vi "Test CAN Flatten.vi"() -> ()   [LabVIEW 2021]
uses:
  typedef/Datatype CAN.ctl
  CIFfifo.lvclass
  CIFfifo.lvclass/CIFfifo.ctl
  Utilities/Flatten Header.vi
  Flatten/CAN Flatten.vi/be899675-9489-4ae7-9bdb-bbc908cd9623.vi
  Flatten/CAN Flatten.vi/fa4e04b0-1c28-4039-87e0-9391600efeb5.vi
  Flatten/CAN Flatten.vi/24dfac9c-4f7b-471b-adb6-3e40fb284e05.vi
  Accessors/Write Payload Length.vi
  Accessors/Read Header.vi
  Utilities/Unflatten Header.vi
  CIFCore/Common/Utilities/Add Error.vi
  Flatten/CAN Flatten.vi/be899675-9489-4ae7-9bdb-bbc908cd9623.vi/c28b0ead-42ad-4072-80a2-aca7f2bd7ce3.vi
  Flatten/CAN Flatten.vi/fa4e04b0-1c28-4039-87e0-9391600efeb5.vi/c28b0ead-42ad-4072-80a2-aca7f2bd7ce3.vi
  Flatten/CAN Flatten.vi/24dfac9c-4f7b-471b-adb6-3e40fb284e05.vi/c28b0ead-42ad-4072-80a2-aca7f2bd7ce3.vi
  CIFCore/Common/Utilities/Append Error Location.vi
  ChannelCommon.lvlib
panel:
  out "error out":errorcluster
  out "Data":T1[](array[typedef]) {"Tags" format="%.0x"; "payload" format="%x"; "identifier" format="%x"}
  in  "CAN Data":T1[](array[typedef])=[{"payload"=[0, 0, 0, 0, 0, 0, 2, 51], "identifier"=291, "Tags"=0, "Timestamp"=0}, {"payload"=[0, 0, 0, 0, 0, 0, 2, 51], "identifier"=837, "Tags"=0, "Timestamp"=0}] {"Tags" format="%.0x"; "payload" format="%x"; "identifier" format="%x"}
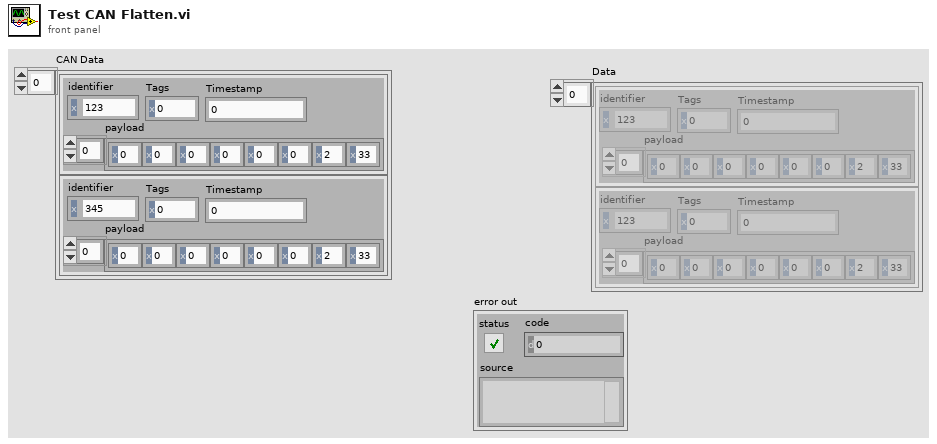
[diagram p1: front panel]
types:
  T1 = typedef "ChannelCommon.lvlib/Datatype CAN.ctl" = cluster{"payload":u8[], "identifier":u32, "Tags":u8, "Timestamp":u64}
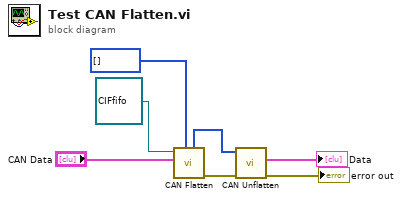
[diagram p0: block diagram]
diagram:
  n1 = call "CAN Flatten.vi"("payload in"=u8[] [], "Data in"="CAN Data", "CIFFifo in"=refnum<class "CIFfifo.lvclass"> refnum) -> ("error out"=w6:errorcluster, "payload out"=w5:u8[])  [unwired: 5 in, 2 out]
  n2 = call "CAN Unflatten.vi"("error in (no error)"=w6, "Flatten Data in"=w5) -> ("error out"=→"error out":errorcluster, "Data"=→"Data":T1[])  [unwired: 6 in, 2 out]
